vi "Find Resource by Type (U32).vi"(6 "Error if not found? (F)":bool, 8 "error in (no error)":errorcluster, 10 "Resource Type":u32, 11 "Resources":T1[](array[typedef])) -> (0 "error out":errorcluster, 1 "Index":i32, 2 "Resource":T1, 3 "Resources out":T1[](array[typedef]), 5 "Found?":bool)   [LabVIEW 2026, in "VILab.lvlib"]
uses:
  VILab.lvlib
  CTLs/Resource.ctl
  <vilib>/Utility/error.llb/Error Cluster From Error Code.vi
  <vilib>/ErrorRing/Error Ring.xnode
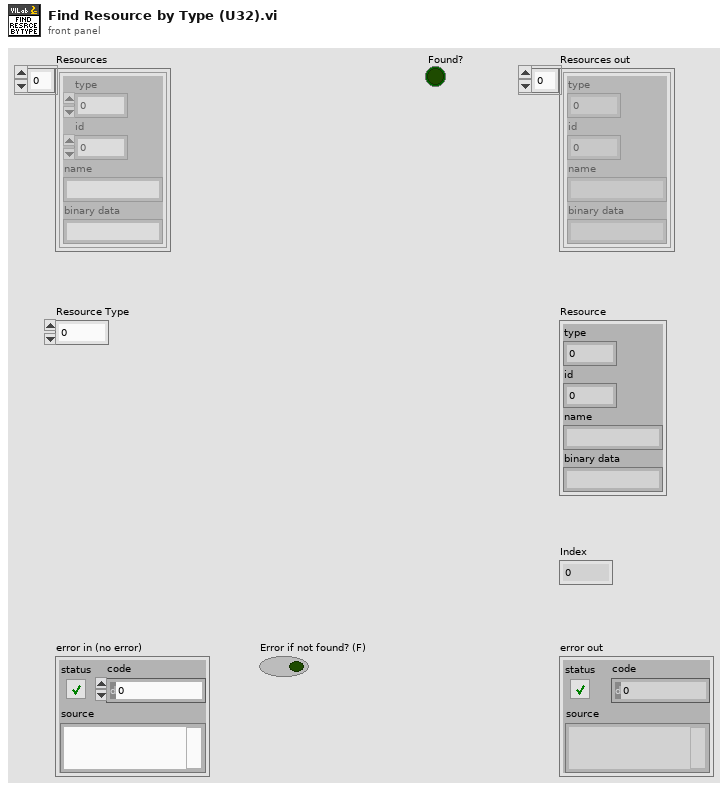
[diagram p1: front panel]
types:
  T1 = typedef "VILab.lvlib/Resource.ctl" = cluster{"type":u32, "id":i32, "name":string, "binary data":string}
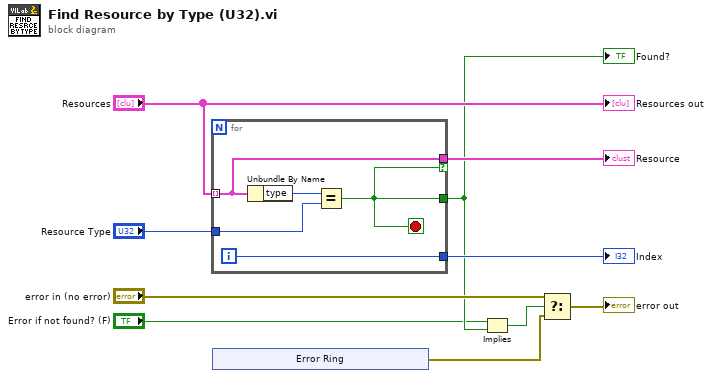
[diagram p0: block diagram]
diagram:
  n1 = for {
    tunnel: "Resources" -> [w13] mode=indexing
    tunnel: "Resource Type" -> [w14]
    tunnel: [w12] -> w5
    tunnel: [w13] -> w7 if=w12
    tunnel: [w11] -> w8
    i -> [w11]
    stop <- w12 stop-if-true
    n2 = Unbundle By Name(w13) -> ("type"=w15:u32)
    n3 = Equal?(x=w15, y=w14) -> (x = y?=w12:bool)
  }
  "Index" <- w8
  "Resource" <- w7
  "Found?" <- w5
  n4 = xnode "Error Ring"() -> ("error out"=w1:errorcluster)
  n5 = Implies(1:w5, 2:"Error if not found? (F)") -> (0:w2:bool)
  n6 = Select(t="error in (no error)", s=w2, f=w1) -> (s? t:f=→"error out":errorcluster)
  "Resources out" <- "Resources"
